vi "DB SPROC No Param.vi"() -> ()   [LabVIEW 2011]
doc: "Executes a stored procedure on the database passed in.\n\n<b>Connection Information</b> - Path to the file DSN for connection to the ODBC database.\n\n<b>Stored Procedure</b> - Name of the stored procedure to execute.\n\n\nVersion 1.0 - 10/20/2009\n\nPhaeron, Inc.\nwww.phaeron.com\ninfo@phaeron.com"
uses:
  <vilib>/addons/database/NI_Database_API.lvlib
  <vilib>/addons/database/_DB Variant To Data/Database Variant To Data.xnode
  <vilib>/addons/database/Connection.llb/DB Tools Open Connec (Path).vi
  <vilib>/addons/database/Connection.llb/Conn Execute.vi
  <vilib>/addons/database/Recordset.llb/Rec Fetch Recordset Data (R).vi
  <vilib>/addons/database/Recordset.llb/Rec Destroy - Connection.vi
panel:
  in  "error in (no error)":errorcluster
  out "error out":errorcluster
  in  "Stored Procedure":string="GetContacts"
  in  "connection information":path=path "SQL.dsn"
  out "Data":string[][](table)
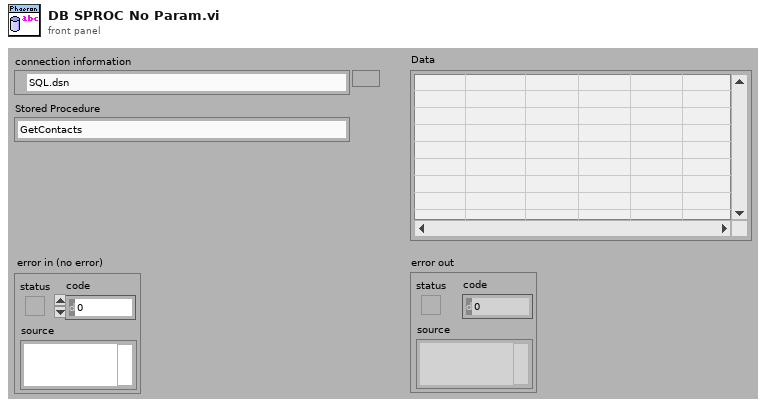
[diagram p1: front panel]
types:
  T1 = typedef "NI_Database_API.lvlib/Conn ObjectReference.ctl" = refnum<k1>
  T2 = typedef "NI_Database_API.lvlib/Rec ObjectReference.ctl" = refnum<k1>
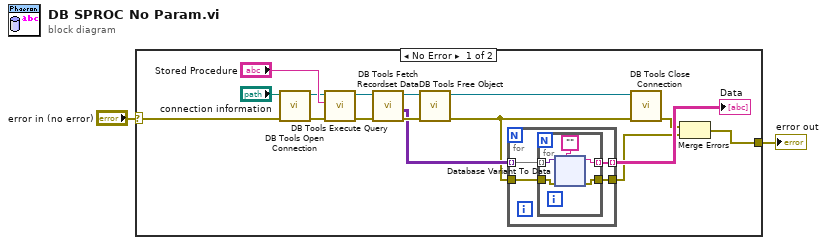
[diagram p0: block diagram]
diagram:
  n1 = case shown="No Error" "error in (no error)" {
    selector: "error in (no error)" -> [w3 w60]
    tunnel: [w11 w60] -> w2
    frame No Error {
      n2 = call-poly <vilib>:"DB Tools Open Connection.vi"("error in (no error)"=w3, "connection information"="connection information") -> ("error out"=w5:errorcluster, "connection reference"=w6:T1)  [unwired: 6 in]
      n3 = call-poly <vilib>:"DB Tools Execute Query.vi"("error in (no error)"=w5, "SQL query"="Stored Procedure", "connection reference"=w6) -> ("error out"=w4:errorcluster, "recordset reference"=w7:T2)  [unwired: 5 in]
      n4 = call-poly <vilib>:"DB Tools Fetch Recordset Data.vi"("error in (no error)"=w4, "recordset reference"=w7) -> ("error out"=w16:errorcluster, "recordset data"=w14:variant[][], "recordset reference out"=w17:T2)  [unwired: 3 in]
      n5 = call-poly <vilib>:"DB Tools Free Object.vi"("error in (no error)"=w16, "recordset reference"=w17) -> ("error out"=w9:errorcluster, "connection reference"=w8:T1)  [unwired: 8 in]
      n6 = for {
        tunnel: [w22] -> w15 mode=indexing
        tunnel: w14 -> [w21] mode=indexing
        tunnel: w9 -> [w20]
        tunnel: [w19] -> w12
        n7 = for {
          tunnel: [w26] -> w22 mode=indexing
          tunnel: w21 -> [w25] mode=indexing
          tunnel: w20 -> [w24]
          tunnel: [w23] -> w19
          n8 = xnode "Database Variant To Data"("database variant"=w25, "error in"=w24, "type"="") -> ("data"=w26:string, "error out"=w23:errorcluster)
        }
      }
      "Data" <- w15
      n9 = call <vilib>:"DB Tools Close Connection.vi"("error in (no error)"=w9, "connection reference"=w8) -> ("error out"=w13:errorcluster)  [unwired: 5 in]
      n10 = Merge Errors(w13, w12) -> (w11:errorcluster)
    }
    frame Error {
    }
  }
  "error out" <- w2
